vi "Configure Math (Binary Operation).vi"(0 "VISA resource name":refnum<visa-resource-name>, 1 "Enable Math Channel (T:Enable)":bool=TRUE, 2 "Math Operation (12: Add)":u16(ring)=12 items=["Add"=12, "Divide"=13, "Multiply"=14, "Subtract"=15, "Common Mode"=16, "Versus"=17], 5 "Math Channel (5: Function 1)":u16(ring)=5 items=["Function 1"=5, "Function 2"=6, "Function 3"=7, "Function 4"=8], 7 "Math Operand (1: Channel 1)":u16(ring)=1 items=["Channel 1"=1, "Channel 2"=2, "Channel 3"=3, "Channel 4"=4, "Function 1"=5, "Function 2"=6, "Function 3"=7, "Function 4"=8, "Memory 1"=9, "Memory 2"=10, "Memory 3"=11, "Memory 4"=12], 9 "Math Operand (2: Channel 2)":u16(ring)=2 items=["Channel 1"=1, "Channel 2"=2, "Channel 3"=3, "Channel 4"=4, "Function 1"=5, "Function 2"=6, "Function 3"=7, "Function 4"=8, "Memory 1"=9, "Memory 2"=10, "Memory 3"=11, "Memory 4"=12], 11 "error in (no error)":errorcluster) -> (4 "VISA resource name out":refnum<visa-resource-name>, 15 "error out":errorcluster)   [LabVIEW 2012, in "Agilent 8000 Series.lvlib"]
doc: "Creates a mathematical expression with two operands."
uses:
  <instrlib>/Agilent 8000 Series/Agilent 8000 Series.lvlib
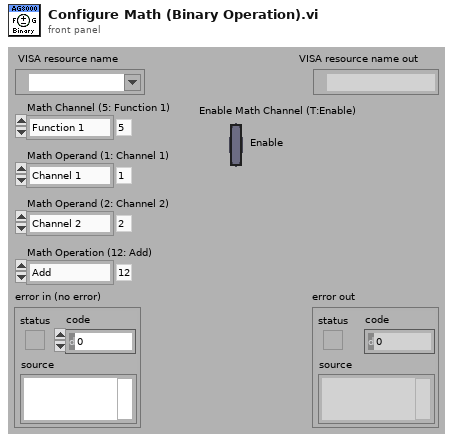
[diagram p1: front panel]
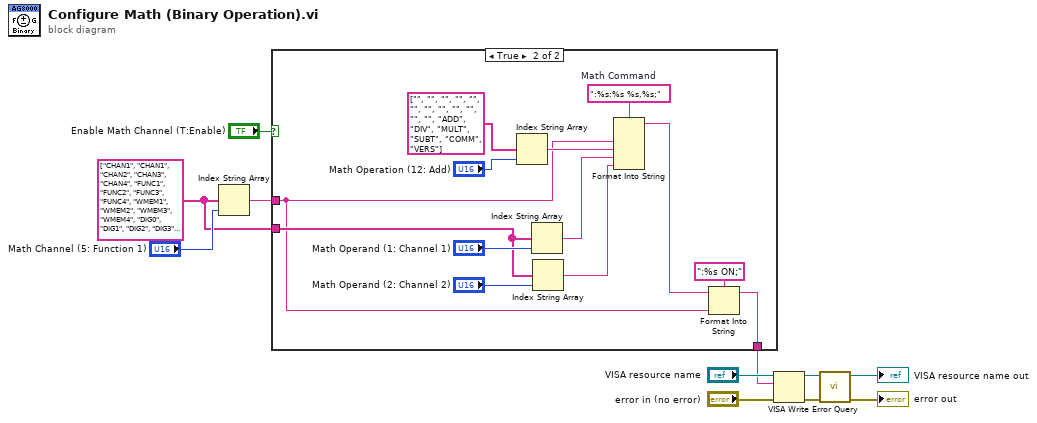
[diagram p0: block diagram]
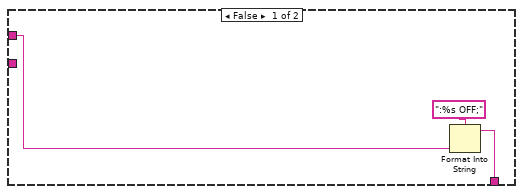
[diagram p2: hidden frame]
diagram:
  w2 = string[] ["CHAN1", "CHAN1", "CHAN2", "CHAN3", "CHAN4", "FUNC1", "FUNC2", "FUNC3", "FUNC4", "WMEM1", "WMEM2", "WMEM3", "WMEM4", "DIG0", "DIG1", "DIG2", "DIG3", "DIG4", "DIG5", "DIG6", "DIG7", "DIG8", "DIG9", "DIG10", "DIG11", "DIG12", "DIG13", "DIG14", "DIG15", "AUX", "LINE"]
  n1 = Index String Array(1:"Math Channel (5: Function 1)", 2:w2) -> (0:w3:string)  [unwired: 1 in]
  n2 = case shown="True" "Enable Math Channel (T:Enable)" {
    tunnel: w3 -> [w13 w16]
    tunnel: w2 -> [_ w19]
    tunnel: [w12 w15] -> w1
    frame False {
      n3 = Format Into String(format string=":%s OFF;", w13) -> (resulting string=w12:string)  [unwired: 2 in, 1 out]
    }
    frame True {
      w26 = ":%s:%s %s,%s;"  # Math Command
      n4 = Index String Array(1:"Math Operation (12: Add)", 2:string[] ["", "", "", "", "", "", "", "", "", "", "", "", "ADD", "DIV", "MULT", "SUBT", "COMM", "VERS"]) -> (0:w25:string)  [unwired: 1 in]
      n5 = Index String Array(1:"Math Operand (1: Channel 1)", 2:w19) -> (0:w21:string)  [unwired: 1 in]
      n6 = Index String Array(1:"Math Operand (2: Channel 2)", 2:w19) -> (0:w20:string)  [unwired: 1 in]
      n7 = Format Into String(format string=w26, w16, w25, w21, w20) -> (resulting string=w17:string)  [unwired: 2 in, 1 out]
      n8 = Format Into String(format string=":%s ON;", initial string=w17, w16) -> (resulting string=w15:string)  [unwired: 1 in, 1 out]
    }
  }
  n9 = VISA Write(VISA resource name="VISA resource name", write buffer=w1, error in (no error)="error in (no error)") -> (VISA resource name out=w7:refnum<visa-resource-name>, error out=w6:errorcluster)  [unwired: 1 out]
  n10 = call <instrlib>:"Error Query.vi"("error in (no error)"=w6, "VISA resource name"=w7) -> ("error out"=→"error out":errorcluster, "VISA resource name out"=→"VISA resource name out":refnum<visa-resource-name>)  [unwired: 6 in, 2 out]
